vi "smart invert.vi"() -> ()   [LabVIEW 2020]
uses:
  <vilib>/Analysis/coordinate.llb/Angle Units.ctl
  <vilib>/Analysis/coordinate.llb/Absolute Angle Difference (scalar).vi
  <vilib>/Analysis/coordinate.llb/Wrap Angle (scalar).vi
  <vilib>/Analysis/coordinate.llb/Set Angle Unit.vi
  <vilib>/Analysis/NI_AAL_Angle.lvlib
panel:
  out "rot out":dbl
  in  "Current Rotation Degrees":dbl
  out "Azimuth Setpoint":dbl
  out "Drive Out":dbl
  in  "Drive In":dbl
  in  "Desired Rotation Degrees":dbl
  # "encoder reads 990"
  # "requested rotation is 45 degrees"
  # "990 mod 360 = 2, remainder 270"
  # "45 degrees = 225 degrees"
  # "so we either want 720-45 or 720+225"
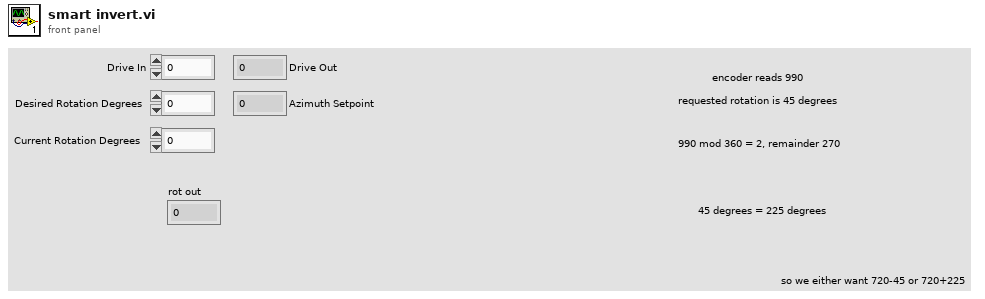
[diagram p1: front panel]
types:
  T1 = typedef "NI_AAL_Angle.lvlib/Angle Units.ctl" = i32
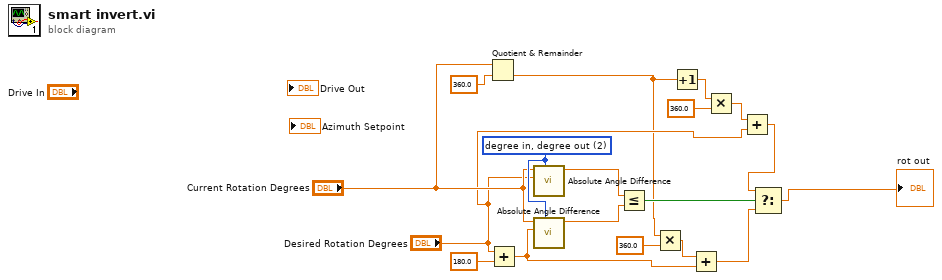
[diagram p0: block diagram]
diagram:
  w18 = T1 2 items=["radian in, radian out", "radian in, degree out", "degree in, degree out", "degree in, radian out"] ("angle units")
  n1 = Quotient & Remainder(x="Current Rotation Degrees", y=360.0) -> (floor(x/y)=w2:dbl)  [unwired: 1 out]
  n2 = Add(x="Desired Rotation Degrees", y=180.0) -> (x+y=w9:dbl)
  n3 = call-poly <vilib>:"Absolute Angle Difference.vi"("angle units"=w18, "angle 2"="Desired Rotation Degrees", "angle 1"="Current Rotation Degrees") -> ("absolute angle difference"=w16:dbl)  [unwired: 7 in, 1 out]
  n4 = call-poly <vilib>:"Absolute Angle Difference.vi"("angle units"=w18, "angle 2"=w9, "angle 1"="Current Rotation Degrees") -> ("absolute angle difference"=w15:dbl)  [unwired: 7 in, 1 out]
  n5 = Less Or Equal?(x=w16, y=w15) -> (x <= y?=w14:bool)
  n6 = Multiply(x=w2, y=360.0) -> (x*y=w11:dbl)
  n7 = Increment(x=w2) -> (x+1=w1:dbl)
  n8 = Add(x=w11, y=w9) -> (x+y=w8:dbl)
  n9 = Multiply(x=w1, y=360.0) -> (x*y=w7:dbl)
  n10 = Add(x=w7, y="Desired Rotation Degrees") -> (x+y=w4:dbl)
  n11 = Select(t=w4, s=w14, f=w8) -> (s? t:f=→"rot out":dbl)
